vi "bit array to number.vi"(10 "bit array":u8[](array[numeric])) -> (2 "Numeric":i32)   [LabVIEW 2014]
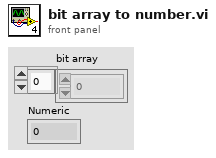
[diagram p1: front panel]
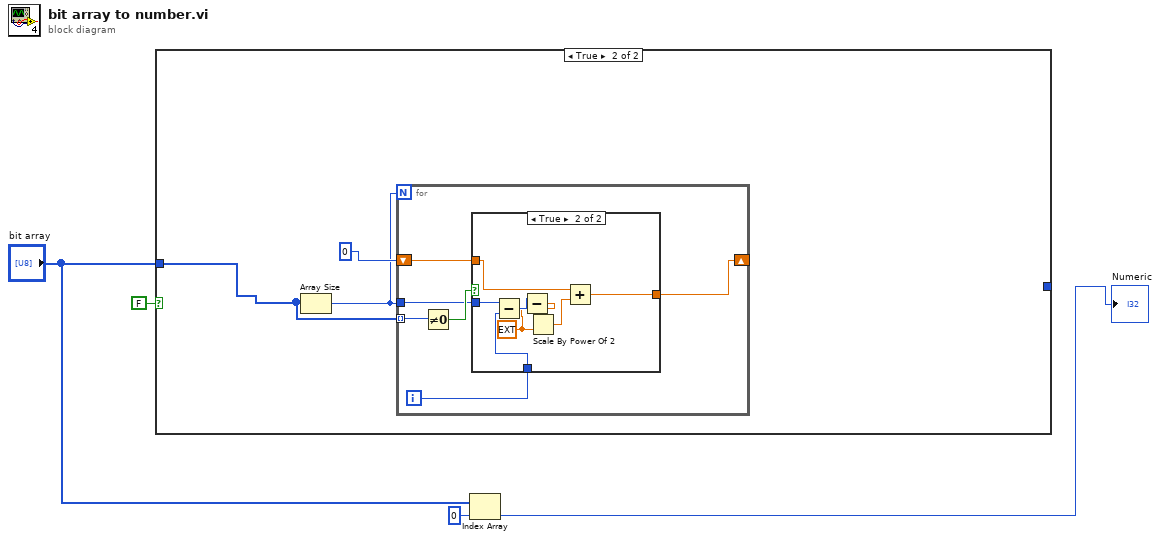
[diagram p0: block diagram]
diagram:
  n1 = case shown="True" FALSE {
    tunnel: "bit array" -> [w5 w6]
    tunnel: [w5 _] -> _
    frame False {
    }
    frame True {
      n2 = Array Size(array=w6) -> (size(s)=w7:i32)
      n3 = for {
        N: w7 -> [_]
        tunnel: w6 -> [w14] mode=indexing
        shift-right: [w10] -> _
        shift-left: 0 -> [w11]
        tunnel: w7 -> [w9]
        i -> [w12]
        n4 = Not Equal To 0?(x=w14) -> (x != 0?=w13:bool)
        n5 = case shown="True" w13 {
          tunnel: w12 -> [_ w19]
          tunnel: w11 -> [w15 w22]
          tunnel: [w15 w21] -> w10
          tunnel: w9 -> [_ w20]
          frame False {
          }
          frame True {
            w17 = ext 1.0 ("x")
            n6 = Subtract(x=w20, y=w19) -> (x-y=w18:i32)
            n7 = Subtract(x=w18, y=w17) -> (x-y=w16:ext)
            n8 = Scale By Power Of 2(n=w16, x=w17) -> (x*2^n=w23:ext)
            n9 = Add(x=w22, y=w23) -> (x+y=w21:ext)
          }
        }
      }
    }
  }
  n10 = Index Array(array="bit array", index=0) -> (element=→"Numeric":u8)
